vi "ColorGraphWindow_LS1.vi"() -> (11 "Graph":dbl[][](graph))   [LabVIEW 2019]
uses:
  Interface Class/2DGraphSetup.ctl
  2DGraphQData.ctl
  Interface Class/PlotChange.ctl
  <vilib>/Utility/config.llb/Read Key (String).vi
  <vilib>/Utility/config.llb/NI_LVConfig.lvlib
panel:
  out "Goto Y":dbl
  out "Goto X":dbl
  in  "2DGphParam":T1={"ZDataIndex"=-1, "XParIndex"=-1, "YParIndex"=-1, "FillLineFirst"=FALSE, "2DGraphIndex"=0, "XParQ Ref"=refnum, "YParQ Ref"=refnum, "DataQRefs"=[], "CurveName"="", "XparInstrInd"=-1, "YparInstrInd"=-1, "Active"=FALSE}
  in  "Goto Active":bool
  out "RéfMenu":refnum<k9>
  out "XY":cluster{"X":dbl, "Y":dbl}
  in  "GraphQRef":refnum<queue>
  in  "MainGraphQ":refnum<queue>
  in  "Graph Event":refnum<user-event>
  in  "ToolsVis":bool
  in  "stop":bool
  out "error out":errorcluster caption="sortie d'erreur"
  in  "error in (no error)":errorcluster
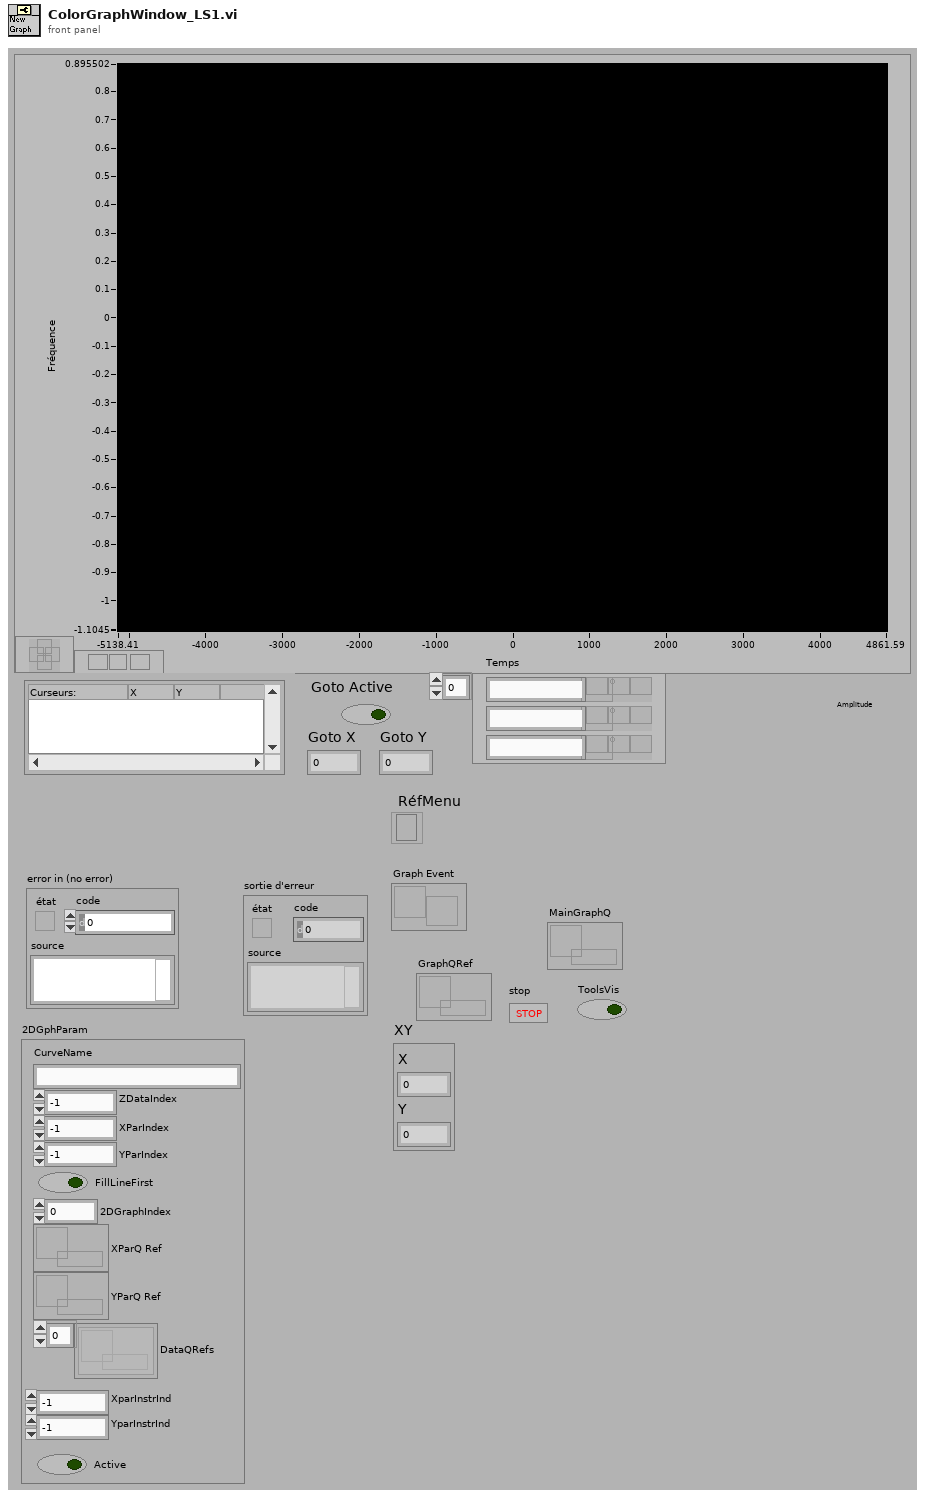
[diagram p1: front panel]
types:
  T1 = typedef "2DGraphSetup.ctl" = cluster{"ZDataIndex":i32, "XParIndex":i32, "YParIndex":i32, "FillLineFirst":bool, "2DGraphIndex":i32, "XParQ Ref":refnum<queue>, "YParQ Ref":refnum<queue>, "DataQRefs":refnum<queue>[], "CurveName":string, "XparInstrInd":i32, "YparInstrInd":i32, "Active":bool}
  T2 = typedef "2DGraphQData.ctl" = cluster{"X Ind(Line)":i32, "Y Ind(Col)":i32, "Data":dbl}
  T3 = enum16{"Répertoire du VI actuel", "Répertoire du parent 1", "Répertoire du parent 2", "Répertoire du parent 3"}
  T4 = cluster{dbl[], "XparInstrInd":i32, "YparInstrInd":i32}
  T5 = typedef "PlotChange.ctl" = cluster{"PlotIdx":i32, "PlotAttrib":cluster{"Color":u32, "PointStyle":u8, "LineStyle":u8, "Interp":u8, "LineWidth":u8, "BarPlotStyle":u8, "FillTo":i16, "XScaleIdx":u32, "YScaleIdx":u32, "Anti-Aliased":bool, "LabelFormat":u8, "TransitionType":u8, "TransitionLocation":u8, "DigitalLineStyle":u8}, "GraphId":i32, "Crv Visible":bool}
  T6 = typedef "LVBoundsTypeDef.ctl" = cluster{"Width":u32, "Height":u32}
  T7 = typedef "imagedata.ctl" = cluster{"image type":i32, "image depth":i32, "image":u8[], "mask":u8[], "colors":u32[], "Rectangle":cluster{"left":i16, "top":i16, "right":i16, "bottom":i16}}
  T8 = typedef "LVPoint32TypeDef.ctl" = cluster{"Horizontal":i32, "Vertical":i32}
  T9 = cluster{"Color":u32, "PointStyle":u8, "LineStyle":u8, "Interp":u8, "LineWidth":u8, "BarPlotStyle":u8, "FillTo":i16, "XScaleIdx":u32, "YScaleIdx":u32, "Anti-Aliased":bool, "LabelFormat":u8, "TransitionType":u8, "TransitionLocation":u8, "DigitalLineStyle":u8}
  T10 = typedef "eventsource.ctl" = u32
  T11 = typedef "NI_LVConfig.lvlib/Config Data RefNum.ctl" = refnum<k1>
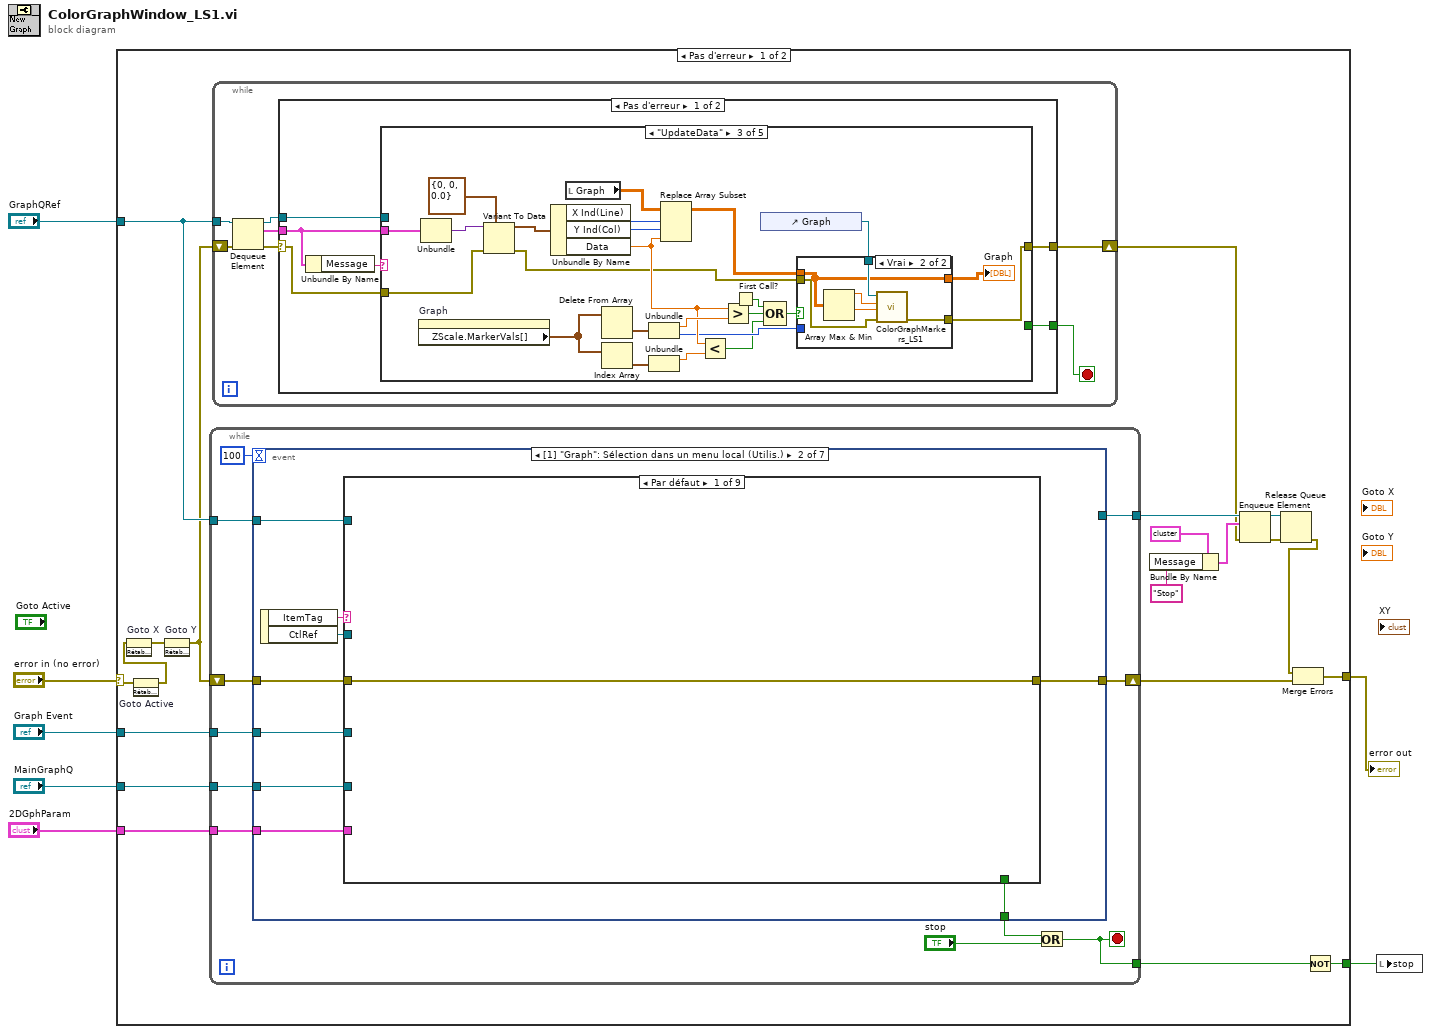
[diagram p0: block diagram]
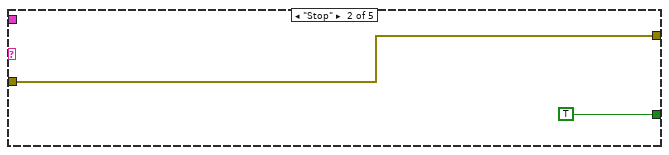
[diagram p3: hidden frame]
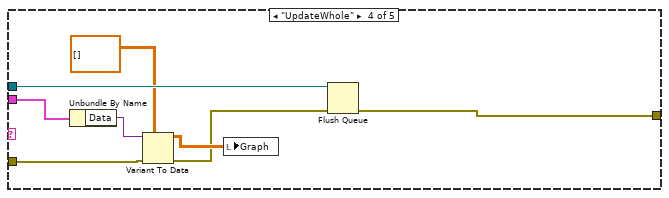
[diagram p5: hidden frame]
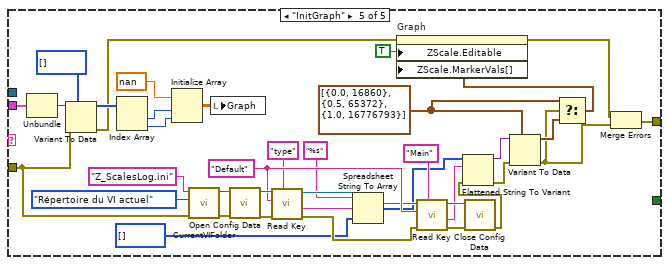
[diagram p6: hidden frame]
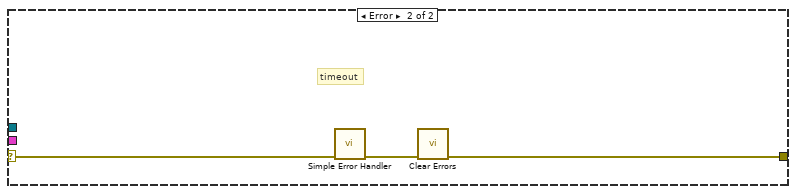
[diagram p7: hidden frame]
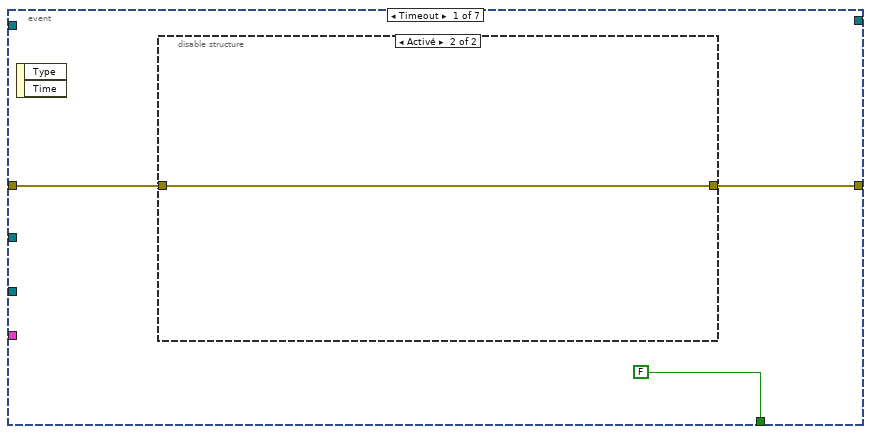
[diagram p8: hidden frame]
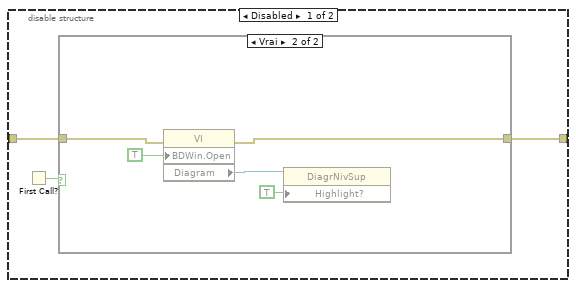
[diagram p9: hidden frame]
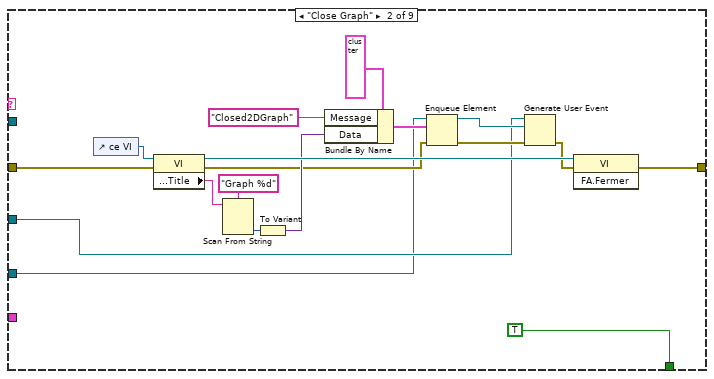
[diagram p11: hidden frame]
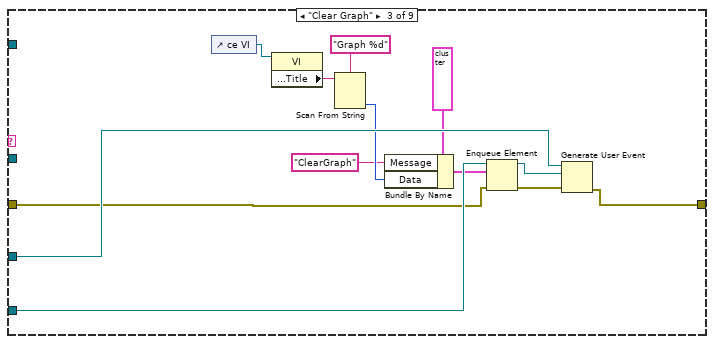
[diagram p12: hidden frame]
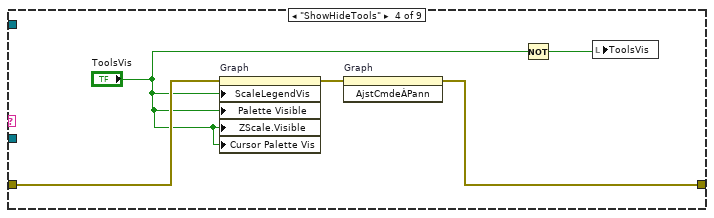
[diagram p13: hidden frame]
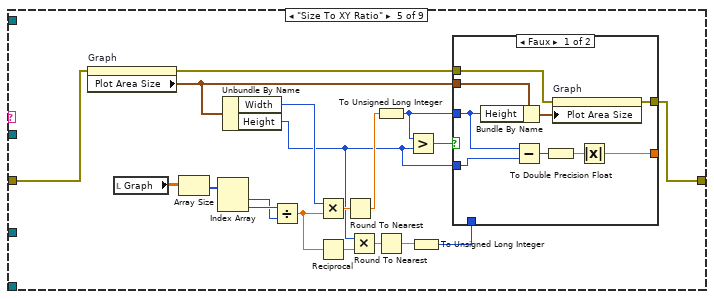
[diagram p14: hidden frame]
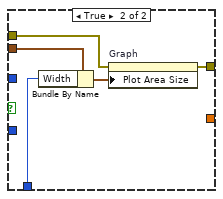
[diagram p15: hidden frame]
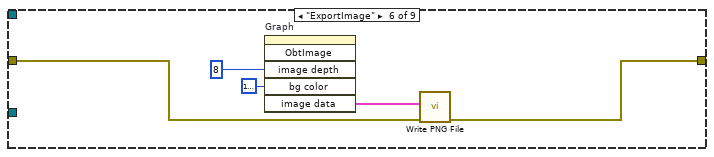
[diagram p16: hidden frame]
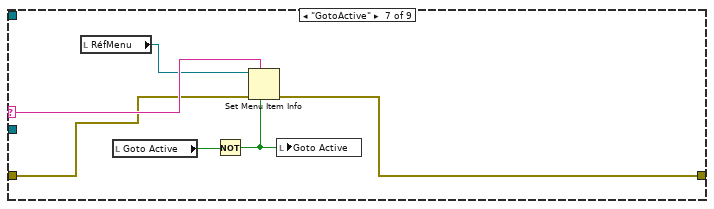
[diagram p17: hidden frame]
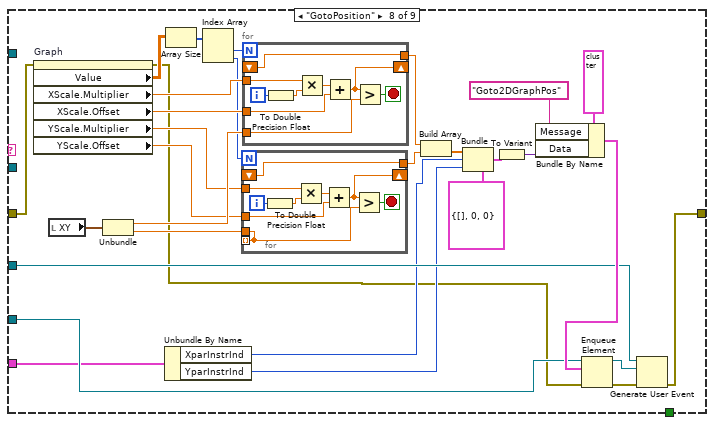
[diagram p18: hidden frame]
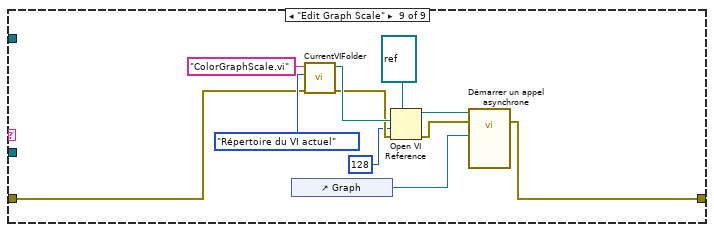
[diagram p19: hidden frame]
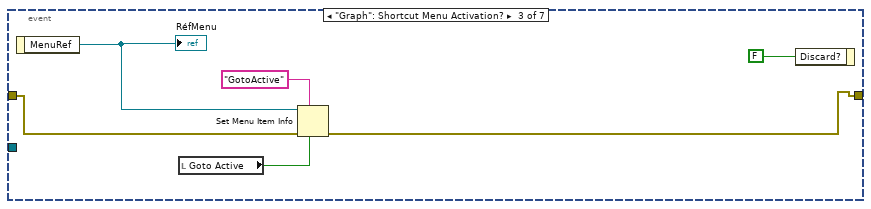
[diagram p20: hidden frame]
diagram:
  n1 = case shown="Pas d'erreur" "error in (no error)" {
    selector: "error in (no error)" -> [w11 w414]
    tunnel: [w20 w414] -> w6
    tunnel: [w26 _] -> w5
    tunnel: "GraphQRef" -> [w24 _]
    tunnel: "Graph Event" -> [w15 _]
    tunnel: "MainGraphQ" -> [w14 _]
    tunnel: "2DGphParam" -> [w12 _]
    frame No Error {
      n2 = invoke on="Goto Active" class="Bool (strict)" method="RétablirValParDéfaut"(error in=w11) -> (error out=w10:errorcluster)  [unwired: 2 in, 2 out]
      n3 = invoke on="Goto X" class="NumNb (strict)" method="RétablirValParDéfaut"(error in=w10) -> (error out=w9:errorcluster)  [unwired: 2 in, 2 out]
      n4 = invoke on="Goto Y" class="NumNb (strict)" method="RétablirValParDéfaut"(error in=w9) -> (error out=w8:errorcluster)  [unwired: 2 in, 2 out]
      n5 = while {
        shift-right: [w132] -> w25
        shift-left: w8 -> [w133]
        tunnel: [w131] -> w27
        tunnel: w24 -> [w130]
        tunnel: [w129] -> w23
        tunnel: w15 -> [w128]
        tunnel: w14 -> [w127]
        tunnel: w12 -> [w125]
        stop <- w131 stop-if-true
        n6 = event shown="[1] \"Graph\": Sélection dans un menu local (Utilis.)" {
          selector: _ -> [_ _ _ _ _ _ _]
          dyn-events: _ -> [_ _ _ _ _ _ _]
          timeout: 100 -> [_ _ _ _ _ _ _]
          tunnel: [FALSE w156 _ _ _ _ TRUE] -> w135
          tunnel: w133 -> [w137 w155 w300 w308 w387 _ w410]
          tunnel: [w136 w154 w299 w307 w375 _ w398] -> w132
          tunnel: w130 -> [_ w153 _ _ _ _ w407]
          tunnel: [_ _ _ _ _ _ w407] -> w129
          tunnel: w128 -> [_ w152 _ w305 w376 _ w397]
          tunnel: w127 -> [_ w151 _ w306 w379 _ w396]
          tunnel: w125 -> [_ w149 _ w304 _ _ _]
          event Timeout {
            n7 = event-data() -> ()  [unwired: 1 in, 2 out]
            n8 = disable-structure shown="Activé" {
              disable-tunnel: w137 -> [w141 w148]
              disable-tunnel: [w140 w148] -> w136
              frame Disabled {
                n9 = First Call?() -> (First Call?: T/F=w139:bool)
                n10 = case shown="Vrai" w139 {
                  tunnel: w141 -> [w142 w146]
                  tunnel: [w142 w145] -> w140
                  frame False {
                  }
                  frame True {
                    n11 = property class="VI"(error in=w146, "BDWin.Open"=TRUE ("Fenêtre du diagramme : ouverte")) -> (error out=w145:errorcluster, "Diagram"=w144:refnum<vi>)  [unwired: 1 in, 1 out]
                    n12 = property class="DiagrNivSup"(reference=w144, "Highlight?"=TRUE ("Animer l'exécution ?")) -> ()  [unwired: 1 in, 2 out]
                  }
                }
              }
              frame Enabled {
              }
            }
          }
          event "Graph": Shortcut Menu Selection (User) {
            n13 = event-data() -> ("ItemTag"=w157:string, "CtlRef"=w150:refnum<vi>)  [unwired: 1 in]
            n14 = case shown="Par défaut" w157 {
              selector: w157 -> [_ _ _ _ _ _ w238 _ _]
              tunnel: [_ TRUE _ _ _ _ _ _ _] -> w156
              tunnel: w155 -> [w158 w171 w185 w193 w203 w231 w236 w259 w294]
              tunnel: [w158 w170 w184 w192 w204 w230 w237 w261 w287] -> w154
              tunnel: w153 -> [_ _ _ _ _ _ _ _ _]
              tunnel: w152 -> [_ w163 w187 _ _ _ _ w263 _]
              tunnel: w151 -> [_ w159 w186 _ _ _ _ w262 _]
              tunnel: w150 -> [_ _ _ _ _ _ _ _ _]
              tunnel: w149 -> [_ _ _ _ _ _ _ w243 _]
              frame Default {
              }
              frame "Close Graph" {
                n15 = control-ref of="ce VI"() -> (w173:refnum<vi>)
                n16 = property class="VI"(reference=w173, error in=w171) -> (reference out=w172:refnum<vi>, error out=w161:errorcluster, "Front Panel.Title"=w174:string)
                n17 = Scan From String(format string="Graph %d" ("chaîne de format"), input string=w174) -> (output 1=w169:i32)  [unwired: 3 in, 3 out]
                n18 = To Variant(anything=w169) -> (Variant=w162:variant)
                n19 = Bundle By Name(cluster=cluster{"Message":string, "Data":variant, i32} {"Message"="", "Data"=variant, 0} ("ClassQueue"), "Message"="Closed2DGraph", "Data"=w162) -> (w165:cluster{"Message":string, "Data":variant, i32})
                n20 = Enqueue Element(queue=w159, element=w165, error in (no error)=w161) -> (queue out=w167:refnum<queue>, error out=w168:errorcluster)  [unwired: 1 in, 1 out]
                n21 = Generate User Event(user event=w163, event data cluster=w167, error in=w168) -> (error out=w160:errorcluster)  [unwired: 1 in, 1 out]
                n22 = invoke class="VI" method="FA.Fermer"(reference=w172, error in=w160) -> (error out=w170:errorcluster)  [unwired: 1 in, 2 out]
              }
              frame "Clear Graph" {
                n23 = control-ref of="ce VI"() -> (w179:refnum<vi>)
                n24 = property class="VI"(reference=w179) -> ("Front Panel.Title"=w180:string)  [unwired: 1 in, 2 out]
                n25 = Scan From String(format string="Graph %d" ("chaîne de format"), input string=w180) -> (output 1=w178:i32)  [unwired: 3 in, 3 out]
                n26 = Bundle By Name(cluster=cluster{"Message":string, "Data":variant, i32} {"Message"="", "Data"=variant, 0} ("ClassQueue"), "Message"="ClearGraph", "Data"=w178) -> (w182:cluster{"Message":string, "Data":variant, i32})
                n27 = Enqueue Element(queue=w186, element=w182, error in (no error)=w185) -> (queue out=w188:refnum<queue>, error out=w189:errorcluster)  [unwired: 1 in, 1 out]
                n28 = Generate User Event(user event=w187, event data cluster=w188, error in=w189) -> (error out=w184:errorcluster)  [unwired: 1 in, 1 out]
              }
              frame "ShowHideTools" {
                n29 = property on="Graph" class="GraphInt (strict)"(error in=w193, "ScaleLegendVis"="ToolsVis", "Palette Visible"="ToolsVis", "ZScale.Visible"="ToolsVis", "Cursor Palette Vis"="ToolsVis") -> (error out=w191:errorcluster)  [unwired: 1 in, 1 out]
                n30 = invoke on="Graph" class="GraphInt (strict)" method="AjstCmdeÀPann"(error in=w191) -> (error out=w192:errorcluster)  [unwired: 2 in, 2 out]
                n31 = Not(x="ToolsVis") -> (.not. x?=w194:bool)
                n32 = local write "ToolsVis"(w194) -> ()
              }
              frame "Size To XY Ratio" {
                n33 = property on="Graph" class="GraphInt (strict)"(error in=w203) -> (error out=w205:errorcluster, "Plot Area Size"=w206:T6)  [unwired: 1 in, 1 out]
                n34 = local read "Graph"() -> (w208:dbl[][])
                n35 = Array Size(array=w208) -> (size(s)=w213:i32[])
                n36 = Index Array(array=w213) -> (element #1=w211:i32, element #2=w212:i32)  [unwired: 2 in]
                n37 = Unbundle By Name(w206) -> ("Width"=w210:u32, "Height"=w195:u32)
                n38 = Divide(x=w212, y=w211) -> (x/y=w200:dbl)
                n39 = Multiply(x=w210, y=w200) -> (x*y=w209:dbl)
                n40 = Reciprocal(x=w200) -> (1/x=w198:dbl)
                n41 = Round To Nearest(number=w209) -> (nearest integer value=w207:dbl)
                n42 = Multiply(x=w195, y=w198) -> (x*y=w199:dbl)
                n43 = To Unsigned Long Integer(number=w207) -> (unsigned 32bit integer=w202:u32)
                n44 = Round To Nearest(number=w199) -> (nearest integer value=w197:dbl)
                n45 = Greater?(x=w202, y=w195) -> (0:w201:bool)
                n46 = To Unsigned Long Integer(number=w197) -> (unsigned 32bit integer=w196:u32)
                n47 = case shown="Faux" w201 {
                  tunnel: w206 -> [w221 w226]
                  tunnel: w205 -> [w220 w225]
                  tunnel: [w219 w224] -> w204
                  tunnel: w202 -> [w218 _]
                  tunnel: w196 -> [_ w223]
                  tunnel: w195 -> [w217 _]
                  tunnel: [w214 _] -> _
                  frame False {
                    n48 = Bundle By Name(cluster=w221, "Height"=w218) -> (w222:T6)
                    n49 = Subtract(x=w218, y=w217) -> (x-y=w216:u32)
                    n50 = To Double Precision Float(number=w216) -> (double precision float=w215:dbl)
                    n51 = property on="Graph" class="GraphInt (strict)"(error in=w220, "Plot Area Size"=w222) -> (error out=w219:errorcluster)  [unwired: 1 in, 1 out]
                    n52 = Absolute Value(x=w215) -> (abs(x)=w214:dbl)
                  }
                  frame True {
                    n53 = Bundle By Name(cluster=w226, "Width"=w223) -> (w227:T6)
                    n54 = property on="Graph" class="GraphInt (strict)"(error in=w225, "Plot Area Size"=w227) -> (error out=w224:errorcluster)  [unwired: 1 in, 1 out]
                  }
                }
              }
              frame "ExportImage" {
                n55 = invoke on="Graph" class="GraphInt (strict)" method="ObtImage"("image depth"=8 ("Profondeur d'image"), "bg color"=u32 16777226 ("Couleur de l'arrière-plan")) -> ("image data"=w232:T7)  [unwired: 4 in, 5 out]
                n56 = call <vilib>:"Write PNG File.vi"("error in (no error)"=w231, "image data"=w232) -> ("error out"=w230:errorcluster)  [unwired: 8 in, 1 out]
              }
              frame "GotoActive" {
                n57 = local read "RéfMenu"() -> (w233:refnum<k9>)
                n58 = local read "Goto Active"() -> (w235:bool)
                n59 = Not(x=w235) -> (.not. x?=w234:bool)
                n60 = Set Menu Item Info(6:w234, 7:w238, 8:w236, 11:w233) -> (0:w237:errorcluster)  [unwired: 3 in, 1 out]
                n61 = local write "Goto Active"(w234) -> ()
              }
              frame "GotoPosition" {
                n62 = property on="Graph" class="GraphInt (strict)"(error in=w259) -> (error out=w239:errorcluster, "Value"=w258:dbl[][], "XScale.Multiplier"=w255:dbl, "XScale.Offset"=w254:dbl, "YScale.Multiplier"=w251:dbl, "YScale.Offset"=w249:dbl)  [unwired: 1 in, 1 out]
                n63 = local read "XY"() -> (w260:cluster{"X":dbl, "Y":dbl})
                n64 = Unbundle(w260) -> ("X"=w253:dbl, "Y"=w250:dbl)
                n65 = Unbundle By Name(w243) -> ("XparInstrInd"=w242:i32, "YparInstrInd"=w241:i32)
                n66 = Array Size(array=w258) -> (size(s)=w257:i32[])
                n67 = Index Array(array=w257) -> (element #1=w256:i32, element #2=w252:i32)  [unwired: 2 in]
                n68 = for {
                  N: w252 -> [_]
                  tunnel: w251 -> [w275]
                  tunnel: w249 -> [w273]
                  tunnel: [w269] -> _ mode=indexing
                  shift-right: [w271] -> _
                  shift-left: _ -> [w270]
                  tunnel: [w270] -> w247
                  tunnel: w250 -> [w269]
                  i -> [w277]
                  stop <- w272 stop-if-true
                  n69 = To Double Precision Float(number=w277) -> (double precision float=w276:dbl)
                  n70 = Multiply(x=w275, y=w276) -> (x*y=w274:dbl)
                  n71 = Add(x=w274, y=w273) -> (x+y=w271:dbl)
                  n72 = Greater?(x=w271, y=w269) -> (0:w272:bool)
                }
                n73 = for {
                  N: w256 -> [_]
                  tunnel: w255 -> [w284]
                  tunnel: w254 -> [w282]
                  tunnel: w253 -> [w281]
                  shift-right: [w279] -> _
                  shift-left: _ -> [w278]
                  tunnel: [w278] -> w248
                  i -> [w286]
                  stop <- w280 stop-if-true
                  n74 = To Double Precision Float(number=w286) -> (double precision float=w285:dbl)
                  n75 = Multiply(x=w284, y=w285) -> (x*y=w283:dbl)
                  n76 = Add(x=w283, y=w282) -> (x+y=w279:dbl)
                  n77 = Greater?(x=w279, y=w281) -> (0:w280:bool)
                }
                n78 = Build Array(w248, w247) -> (w244:dbl[])
                n79 = Bundle(cluster=T4 {[], "XparInstrInd"=0, "YparInstrInd"=0}, w244, "XparInstrInd"=w242, "YparInstrInd"=w241) -> (w246:T4)
                n80 = To Variant(anything=w246) -> (Variant=w245:variant)
                n81 = Bundle By Name(cluster=cluster{"Message":string, "Data":variant, i32} {"Message"="", "Data"=variant, 0} ("ClassQueue"), "Message"="Goto2DGraphPos", "Data"=w245) -> (w265:cluster{"Message":string, "Data":variant, i32})
                n82 = Enqueue Element(queue=w262, element=w265, error in (no error)=w239) -> (queue out=w267:refnum<queue>, error out=w268:errorcluster)  [unwired: 1 in, 1 out]
                n83 = Generate User Event(user event=w263, event data cluster=w267, error in=w268) -> (error out=w261:errorcluster)  [unwired: 1 in, 1 out]
              }
              frame "Edit Graph Scale" {
                n84 = control-ref of="Graph"() -> (w289:refnum<vi>)
                n85 = call <userlib>:"CurrentVIFolder.vi"("error in (no error)"=w294, "Source"=T3."Répertoire du VI actuel", "NomFichier"="ColorGraphScale.vi") -> ("error out"=w292:errorcluster, "Chemin"=w293:path)  [unwired: 6 in, 1 out]
                n86 = Open VI Reference(type specifier VI Refnum (for type only)=refnum<vi> refnum ("spécificateur de type du refnum de VI (pour type seulement)"), vi path=w293, options=128, error in (no error)=w292) -> (vi reference=w297:refnum<vi>, error out=w291:errorcluster)  [unwired: 2 in]
                n87 = call-by-ref "Démarrer un appel asynchrone"(reference=w297, error in=w291, "GraphRef"=w289) -> (error out=w287:errorcluster)  [unwired: 11 in, 1 out]
              }
            }
          }
          event "Graph": Shortcut Menu Activation? {
            n88 = event-data() -> ("MenuRef"=w302:refnum<k9>)  [unwired: 1 in]
            "RéfMenu" <- w302
            n89 = local read "Goto Active"() -> (w298:bool)
            n90 = Set Menu Item Info(6:w298, 7:"GotoActive" ("tag d'élément"), 8:w300, 11:w302) -> (0:w299:errorcluster)  [unwired: 3 in, 1 out]
            n91 = event-data("Discard?"=FALSE ("Rejeter ?")) -> ()  [unwired: 1 in, 1 out]
          }
          event "Graph": Mouse Down {
            n92 = event-data() -> ("Coords"=w310:T8, "Button"=w309:u16)  [unwired: 1 in]
            n93 = case shown="1" w309 {
              tunnel: w310 -> [_ w315 w374]
              tunnel: w308 -> [w311 w316 w373]
              tunnel: [w311 w317 w372] -> w307
              tunnel: w306 -> [_ w314 _]
              tunnel: w305 -> [_ w313 _]
              tunnel: w304 -> [_ w312 _]
              frame 0, Default {
              }
              frame 1 {
                n94 = local read "Goto Active"() -> (w318:bool)
                n95 = case shown="Vrai" w318 {
                  tunnel: [w319 w332] -> w317
                  tunnel: w316 -> [w319 w333]
                  tunnel: w315 -> [_ w334]
                  tunnel: w314 -> [_ w337]
                  tunnel: w313 -> [_ w336]
                  tunnel: w312 -> [_ w324]
                  frame False {
                  }
                  frame True {
                    n96 = property on="Graph" class="GraphInt (strict)"(error in=w333) -> (error out=w331:errorcluster, "Value"=w349:dbl[][], "XScale.Multiplier"=w346:dbl, "XScale.Offset"=w345:dbl, "YScale.Multiplier"=w342:dbl, "YScale.Offset"=w340:dbl)  [unwired: 1 in, 1 out]
                    n97 = invoke on="Graph" class="GraphInt (strict)" method="AssocCoordsÀXY"(error in=w333, "Coords"=w334) -> (error out=w330:errorcluster, "XY"=w335:cluster{"X":dbl, "Y":dbl})  [unwired: 5 in, 5 out]
                    n98 = Array Size(array=w349) -> (size(s)=w348:i32[])
                    n99 = Unbundle(w335) -> ("X"=w344:dbl, "Y"=w341:dbl)
                    n100 = Index Array(array=w348) -> (element #1=w347:i32, element #2=w343:i32)  [unwired: 2 in]
                    n101 = Unbundle By Name(w324) -> ("XparInstrInd"=w323:i32, "YparInstrInd"=w322:i32)
                    n102 = for {
                      N: w343 -> [_]
                      tunnel: w342 -> [w359]
                      tunnel: w340 -> [w357]
                      shift-right: [w355] -> _
                      shift-left: _ -> [w354]
                      tunnel: [w354] -> w320
                      tunnel: w341 -> [w353]
                      i -> [w361]
                      stop <- w356 stop-if-true
                      n103 = To Double Precision Float(number=w361) -> (double precision float=w360:dbl)
                      n104 = Multiply(x=w359, y=w360) -> (x*y=w358:dbl)
                      n105 = Add(x=w358, y=w357) -> (x+y=w355:dbl)
                      n106 = Greater?(x=w355, y=w353) -> (0:w356:bool)
                    }
                    n107 = for {
                      N: w347 -> [_]
                      tunnel: w346 -> [w368]
                      tunnel: w345 -> [w366]
                      tunnel: w344 -> [w365]
                      shift-right: [w363] -> _
                      shift-left: _ -> [w362]
                      tunnel: [w362] -> w321
                      i -> [w370]
                      stop <- w364 stop-if-true
                      n108 = To Double Precision Float(number=w370) -> (double precision float=w369:dbl)
                      n109 = Multiply(x=w368, y=w369) -> (x*y=w367:dbl)
                      n110 = Add(x=w367, y=w366) -> (x+y=w363:dbl)
                      n111 = Greater?(x=w363, y=w365) -> (0:w364:bool)
                    }
                    n112 = Build Array(w321, w320) -> (w327:dbl[])
                    n113 = Bundle(cluster=T4 {[], "XparInstrInd"=0, "YparInstrInd"=0}, w327, "XparInstrInd"=w323, "YparInstrInd"=w322) -> (w326:T4)
                    n114 = local write "Goto X"(w321) -> ()
                    n115 = To Variant(anything=w326) -> (Variant=w328:variant)
                    n116 = Bundle By Name(cluster=cluster{"Message":string, "Data":variant, i32} {"Message"="", "Data"=variant, 0} ("ClassQueue"), "Message"="Goto2DGraphPos", "Data"=w328) -> (w350:cluster{"Message":string, "Data":variant, i32})
                    n117 = Enqueue Element(queue=w337, element=w350, error in (no error)=w330) -> (queue out=w351:refnum<queue>, error out=w352:errorcluster)  [unwired: 1 in, 1 out]
                    n118 = local write "Goto Y"(w320) -> ()
                    n119 = Generate User Event(user event=w336, event data cluster=w351, error in=w352) -> (error out=w329:errorcluster)  [unwired: 1 in, 1 out]
                    n120 = Merge Errors(w331, w329) -> (w332:errorcluster)
                  }
                }
              }
              frame 2 {
                n121 = invoke on="Graph" class="GraphInt (strict)" method="AssocCoordsÀXY"(error in=w373, "Coords"=w374) -> (error out=w372:errorcluster, "XY"=w371:cluster{"X":dbl, "Y":dbl})  [unwired: 5 in, 5 out]
                n122 = local write "XY"(w371) -> ()
              }
            }
          }
          event "Graph": Plot Attribute Change {
            n123 = event-data() -> ("PlotIdx"=w391:i32, "NewAttrib"=w392:T9)  [unwired: 1 in]
            n124 = control-ref of="ce VI"() -> (w388:refnum<vi>)
            n125 = property class="VI"(reference=w388, error in=w387) -> (error out=w381:errorcluster, "Front Panel.Title"=w389:string)  [unwired: 1 out]
            n126 = Scan From String(format string="Graph %d" ("chaîne de format"), input string=w389) -> (output 1=w386:i32)  [unwired: 3 in, 3 out]
            n127 = Bundle By Name(cluster=T5 {"PlotIdx"=0, "PlotAttrib"={"Color"=0, "PointStyle"=0, "LineStyle"=0, "Interp"=0, "LineWidth"=0, "BarPlotStyle"=0, "FillTo"=0, "XScaleIdx"=0, "YScaleIdx"=0, "Anti-Aliased"=FALSE, "LabelFormat"=0, "TransitionType"=0, "TransitionLocation"=0, "DigitalLineStyle"=0}, "GraphId"=0, "Crv Visible"=FALSE} ("Valeur"), "GraphId"=w386, "PlotIdx"=w391, "PlotAttrib"=w392) -> (w385:T5)
            n128 = To Variant(anything=w385) -> (Variant=w380:variant)
            n129 = Bundle By Name(cluster=cluster{"Message":string, "Data":variant, i32} {"Message"="", "Data"=variant, 0} ("ClassQueue"), "Message"="PlotChange", "Data"=w380) -> (w378:cluster{"Message":string, "Data":variant, i32})
            n130 = Enqueue Element(queue=w379, element=w378, error in (no error)=w381) -> (queue out=w383:refnum<queue>, error out=w384:errorcluster)  [unwired: 1 in, 1 out]
            n131 = Generate User Event(user event=w376, event data cluster=w383, error in=w384) -> (error out=w375:errorcluster)  [unwired: 1 in, 1 out]
          }
          event "Graph": Scale Range Change {
            n132 = event-data() -> ("Source"=w395:T10, "ScaleRef"=w394:refnum<vi>)  [unwired: 1 in, 6 out]
            n133 = flat-sequence {
              tunnel: w395 -> [_]
              tunnel: w394 -> [_]
              frame #0 {
              }
            }
          }
          event Panel Close? {
            n134 = event-data() -> ()  [unwired: 1 in, 1 out]
            n135 = control-ref of="ce VI"() -> (w411:refnum<vi>)
            n136 = property class="VI"(reference=w411, error in=w410) -> (error out=w399:errorcluster, "Front Panel.Title"=w412:string)  [unwired: 1 out]
            n137 = Scan From String(format string="Graph %d" ("chaîne de format"), input string=w412) -> (output 1=w400:i32)  [unwired: 3 in, 3 out]
            n138 = To Variant(anything=w400) -> (Variant=w403:variant)
            n139 = Bundle By Name(cluster=cluster{"Message":string, "Data":variant, i32} {"Message"="", "Data"=variant, 0} ("ClassQueue"), "Message"="Closed2DGraph", "Data"=w403) -> (w402:cluster{"Message":string, "Data":variant, i32})
            n140 = Enqueue Element(queue=w396, element=w402, error in (no error)=w399) -> (queue out=w405:refnum<queue>, error out=w406:errorcluster)  [unwired: 1 in, 1 out]
            n141 = Generate User Event(user event=w397, event data cluster=w405, error in=w406) -> (error out=w398:errorcluster)  [unwired: 1 in, 1 out]
            n142 = event-data("Discard?"=FALSE ("Rejeter ?")) -> ()  [unwired: 1 in, 1 out]
          }
        }
        n143 = Or(x=w135, y="stop") -> (x .or. y?=w131:bool)
      }
      n144 = while {
        tunnel: w24 -> [w34]
        shift-right: [w31] -> w19
        shift-left: w8 -> [w32]
        stop <- w29 stop-if-true
        n145 = Dequeue Element(queue=w34, error in (no error)=w32) -> (queue out=w28:refnum<queue>, element=w30:cluster{"Message":string, "Data":variant, i32}, error out=w33:errorcluster)  [unwired: 1 in, 1 out]
        n146 = case shown="Pas d'erreur" w33 {
          selector: w33 -> [w40 w124]
          tunnel: [w36 w122] -> w31
          tunnel: w30 -> [w39 _]
          tunnel: [w37 _] -> w29
          tunnel: w28 -> [w35 _]
          frame No Error {
            n147 = Unbundle By Name(w39) -> ("Message"=w38:string)
            n148 = case shown="\"UpdateData\"" w38 {
              tunnel: w39 -> [_ _ w67 w81 w121]
              tunnel: [w41 w43 w44 w83 w96] -> w36
              tunnel: w40 -> [w41 w43 w64 w77 w99]
              tunnel: [_ TRUE _ _ _] -> w37
              tunnel: w35 -> [_ _ _ w82 _]
              frame Default {
              }
              frame "Stop" {
              }
              frame "UpdateData" {
                n149 = property on="Graph" class="GraphInt (strict)"() -> ("ZScale.MarkerVals[]"=w57:cluster{dbl, u32}[])  [unwired: 2 in, 2 out]
                n150 = Unbundle(w67) -> ("Data"=w66:variant)  [unwired: 2 out]
                n151 = Variant To Data(error in=w64, type=T2 {"X Ind(Line)"=0, "Y Ind(Col)"=0, "Data"=0.0} ("2DGphQData"), Variant=w66) -> (data=w63:T2, error out=w45:errorcluster)
                n152 = Unbundle By Name(w63) -> ("X Ind(Line)"=w61:i32, "Y Ind(Col)"=w60:i32, "Data"=w53:dbl)
                n153 = local read "Graph"() -> (w62:dbl[][])
                n154 = Delete From Array(array=w57) -> (deleted portion=w54:cluster{dbl, u32})  [unwired: 2 in, 1 out]
                n155 = Index Array(array=w57) -> (element=w59:cluster{dbl, u32})  [unwired: 1 in]
                n156 = Unbundle(w54) -> (w56:dbl, w52:u32)
                n157 = Unbundle(w59) -> (w58:dbl)  [unwired: 1 out]
                n158 = Replace Array Subset(array=w62, new element=w53, index (row)=w61, index (col)=w60) -> (w47:dbl[][])
                n159 = Less?(x=w53, y=w58) -> (x < y?=w50:bool)
                n160 = Greater?(x=w53, y=w56) -> (0:w55:bool)
                n161 = First Call?() -> (First Call?: T/F=w49:bool)
                n162 = control-ref of="Graph"() -> (w48:refnum<vi>)
                n163 = Compound Arithmetic op=OR ("Opérateur arithmétique")(w49, w55, w50) -> (w51:bool)
                n164 = case shown="Vrai" w51 {
                  tunnel: w52 -> [_ _]
                  tunnel: w48 -> [_ w75]
                  tunnel: w47 -> [w69 w74]
                  tunnel: [w69 w74] -> w46
                  tunnel: w45 -> [w68 w71]
                  tunnel: [w68 w70] -> w44
                  frame False {
                  }
                  frame True {
                    n165 = Array Max & Min(array=w74) -> (max value=w73:dbl, min value=w72:dbl)  [unwired: 2 out]
                    n166 = call "ColorGraphMarkers_LS1.vi"("error in (no error)"=w71, "DataMin"=w72, "DataMax"=w73, "GraphRef"=w75) -> ("error out"=w70:errorcluster)  [unwired: 6 in, 1 out]
                  }
                }
                "Graph" <- w46
              }
              frame "UpdateWhole" {
                n167 = Unbundle By Name(w81) -> ("Data"=w80:variant)
                n168 = Variant To Data(error in=w77, type=dbl[][] [] ("Graph"), Variant=w80) -> (data=w78:dbl[][], error out=w76:errorcluster)
                n169 = local write "Graph"(w78) -> ()
                n170 = Flush Queue(queue=w82, error in (no error)=w76) -> (error out=w83:errorcluster)  [unwired: 2 out]
              }
              frame "InitGraph" {
                w100 = "Default"
                w87 = cluster{"MarkerVal":dbl, "ColorVal":u32}[] [{"MarkerVal"=0.0, "ColorVal"=16860}, {"MarkerVal"=0.5, "ColorVal"=65372}, {"MarkerVal"=1.0, "ColorVal"=16776793}] ("Z.MarkVal")
                n171 = Unbundle(w121) -> ("Data"=w120:variant)  [unwired: 2 out]
                n172 = Variant To Data(error in=w99, type=i32[] [], Variant=w120) -> (data=w118:i32[], error out=w112:errorcluster)
                n173 = Index Array(array=w118) -> (element #1=w117:i32, element #2=w115:i32)  [unwired: 2 in]
                n174 = Initialize Array(nan ("élément"), w117, w115) -> (w114:dbl[][])
                n175 = call <userlib>:"CurrentVIFolder.vi"("error in (no error)"=w99, "Source"=T3."Répertoire du VI actuel", "NomFichier"="Z_ScalesLog.ini") -> ("error out"=w108:errorcluster, "Chemin"=w107:path)  [unwired: 6 in, 1 out]
                n176 = local write "Graph"(w114) -> ()
                n177 = call <vilib>:"Open Config Data.vi"("error in (no error)"=w108, "configuration file path"=w107) -> ("error out"=w101:errorcluster, "refnum"=w102:T11)  [unwired: 7 in, 1 out]
                n178 = call-poly <vilib>:"Read Key.vi"("section"="type", "error in (no error)"=w101, "key"=w100, "refnum"=w102) -> ("error out"=w94:errorcluster, "value"=w95:string, "refnum out"=w97:T11)  [unwired: 4 in, 1 out]
                n179 = Spreadsheet String To Array(format string="%s" ("chaîne de format"), spreadsheet string=w95, array type (2D Dbl)=i16[] [] ("chaîne de type")) -> (array=w92:i16[])  [unwired: 1 in]
                n180 = call-poly <vilib>:"Read Key.vi"("section"="Main", "error in (no error)"=w94, "key"=w100, "refnum"=w97) -> ("error out"=w109:errorcluster, "value"=w103:string, "refnum out"=w110:T11)  [unwired: 4 in, 1 out]
                n181 = call <vilib>:"Close Config Data.vi"("error in (no error)"=w109, "refnum"=w110) -> ("error out"=w89:errorcluster)  [unwired: 8 in, 1 out]
                n182 = Flattened String To Variant(4:w89, 6:w103, 7:w92) -> (0:w90:errorcluster, 3:w91:variant)
                n183 = Variant To Data(error in=w90, type=w87, Variant=w91) -> (data=w86:cluster{"MarkerVal":dbl, "ColorVal":u32}[], error out=w84:errorcluster)
                n184 = Select(t=w87, s=w84, f=w86) -> (s? t:f=w85:cluster{"MarkerVal":dbl, "ColorVal":u32}[])
                n185 = property on="Graph" class="GraphInt (strict)"(error in=w112, "ZScale.Editable"=TRUE ("Échelle des Z.Éditable"), "ZScale.MarkerVals[]"=w85) -> (error out=w111:errorcluster)  [unwired: 1 in, 1 out]
                n186 = Merge Errors(w111, w84) -> (w96:errorcluster)
              }
            }
          }
          frame Error {
            # "timeout"
            n187 = call <vilib>:"Simple Error Handler.vi"("error in (no error)"=w124) -> ("error out"=w123:errorcluster)  [unwired: 4 in, 4 out]
            n188 = call <vilib>:"Clear Errors.vi"("error in (no error)"=w123) -> ("error out"=w122:errorcluster)  [unwired: 5 in, 1 out]
          }
        }
      }
      n189 = Bundle By Name(cluster=cluster{"Message":string, "Data":variant, i32} {"Message"="", "Data"=variant, 0} ("élément"), "Message"="Stop") -> (w22:cluster{"Message":string, "Data":variant, i32})
      n190 = Enqueue Element(queue=w23, element=w22, error in (no error)=w19) -> (queue out=w18:refnum<queue>, error out=w17:errorcluster)  [unwired: 1 in, 1 out]
      n191 = Release Queue(queue=w18, error in (no error)=w17) -> (error out=w16:errorcluster)  [unwired: 1 in, 2 out]
      n192 = Merge Errors(w16, w25) -> (w20:errorcluster)
      n193 = Not(x=w27) -> (.not. x?=w26:bool)
    }
    frame Error {
    }
  }
  "error out" <- w6
  n194 = local write "stop"(w5) -> ()
